vi "Close.vi"(8 "error in":errorcluster, 11 "DB-ADO in":refnum<class "DB-ADO.lvclass">) -> (0 "error out":errorcluster, 3 "DB-ADO out":refnum<class "DB-ADO.lvclass">)   [LabVIEW 2014, in "hse-db.lvlib" / "DB-ADO.lvclass"]
doc: "Close the ADO connection."
uses:
  DB-ADO.lvclass
  DB-ADO.lvclass/DB-ADO.ctl
  DB-Engines/ADO-DB-Drivers/ADO-DB-Driver.lvlib
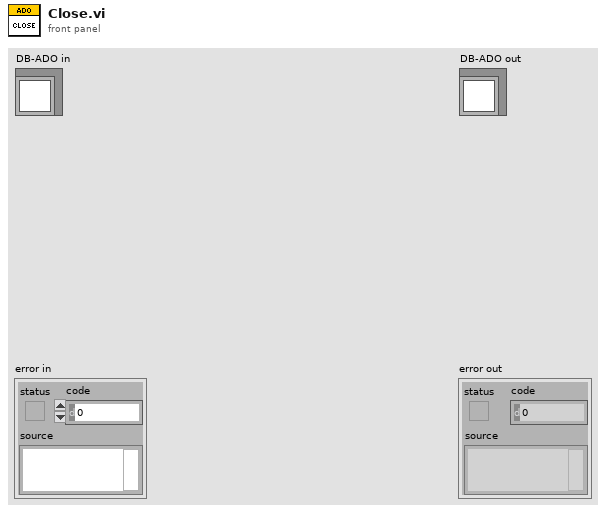
[diagram p1: front panel]
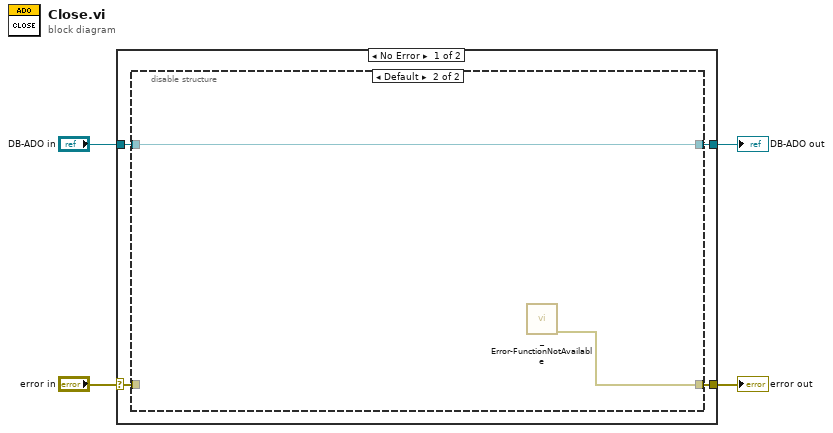
[diagram p0: block diagram]
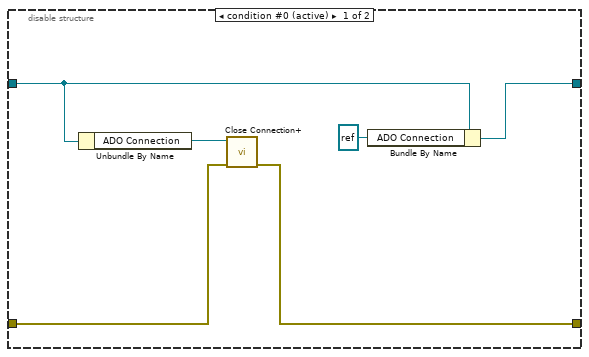
[diagram p2: hidden frame]
diagram:
  n1 = case shown="No Error" "error in" {
    selector: "error in" -> [w8 w18]
    tunnel: [w7 w18] -> w3
    tunnel: [w5 w17] -> w1
    tunnel: "DB-ADO in" -> [w6 w17]
    frame No Error {
      n2 = disable-structure shown="Default" {
        disable-tunnel: w8 -> [w13 _]
        disable-tunnel: [w12 w15] -> w7
        disable-tunnel: w6 -> [w11 w16]
        disable-tunnel: [w10 w16] -> w5
        frame condition #0 (active) {
          n3 = Unbundle By Name(w11) -> ("ADO Connection"=w14:refnum<k7>)
          n4 = call "Close Connection+.vi"("error in"=w13, "Connection"=w14) -> ("error out"=w12:errorcluster)  [unwired: 5 in]
          n5 = Bundle By Name(cluster=w11, "ADO Connection"=refnum<k7> refnum) -> (w10:refnum<class "DB-ADO.lvclass">)
        }
        frame condition #1 {
          n6 = call "_Error-FunctionNotAvailable.vi"() -> ("error out"=w15:errorcluster)  [unwired: 11 in]
        }
      }
    }
    frame Error {
    }
  }
  "error out" <- w3
  "DB-ADO out" <- w1
